vi "p2.vi"() -> ()   [LabVIEW 2023, in "d22.lvlib"]
uses:
  d22.lvlib
  AOC/AOC.lvlib
panel:
  out "size(s)":i32=375
  in  "Example":string="1,0,1~1,2,1\n0,0,2~2,0,2\n0,2,3~2,2,3\n0,0,4~0,2,4\n2,0,5~2,2,5\n0,1,6~2,1,6\n1,1,8~1,1,9"
  in  "Example":bool
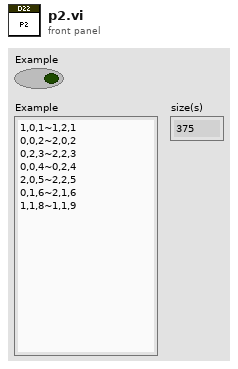
[diagram p1: front panel]
types:
  T1 = cluster{"max":cluster{"x":i32, "y":i32, "z":i32}, "min":cluster{"x":i32, "y":i32, "z":i32}, "supported by":i32[], "supporting":i32[]}
  T2 = cluster{"max":cluster{"x":i32, "y":i32, "z":i32}, "min":cluster{"x":i32, "y":i32, "z":i32}, "supported by":i32[], "supporting":i32[]}[]
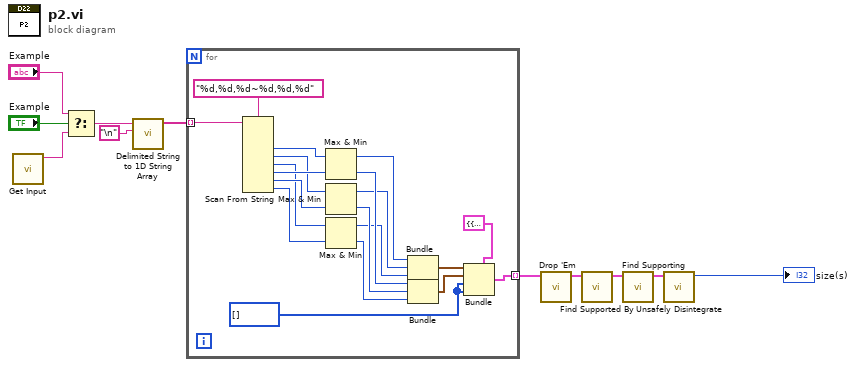
[diagram p0: block diagram]
diagram:
  n1 = call "Get Input.vi"() -> ("Input"=w11:string)  [unwired: 11 in]
  n2 = Select(t="Example", s="Example", f=w11) -> (s? t:f=w10:string)
  n3 = call <vilib>:"Delimited String to 1D String Array.vi"("delimiter"="\n", "delimited string"=w10) -> ("string array"=w7:string[])  [unwired: 9 in]
  n4 = for {
    tunnel: w7 -> [w30] mode=indexing
    tunnel: [w28] -> w6 mode=indexing
    w12 = i32[] [] ("supports")
    n5 = Scan From String(format string="%d,%d,%d~%d,%d,%d", input string=w30) -> (output 1=w26:i32, output 2=w24:i32, output 3=w22:i32, output 4=w25:i32, output 5=w23:i32, output 6=w21:i32)  [unwired: 8 in, 3 out]
    n6 = Max & Min(x=w26, y=w25) -> (max(x,y)=w16:i32, min(x,y)=w17:i32)
    n7 = Max & Min(x=w24, y=w23) -> (max(x,y)=w15:i32, min(x,y)=w18:i32)
    n8 = Max & Min(x=w22, y=w21) -> (max(x,y)=w14:i32, min(x,y)=w19:i32)
    n9 = Bundle(w16, w15, w14) -> (w29:cluster{i32, i32, i32})  [unwired: 1 in]
    n10 = Bundle(w17, w18, w19) -> (w20:cluster{i32, i32, i32})  [unwired: 1 in]
    n11 = Bundle(cluster=T1 {"max"={"x"=0, "y"=0, "z"=0}, "min"={"x"=0, "y"=0, "z"=0}, "supported by"=[], "supporting"=[]}, "max"=w29, "min"=w20, "supported by"=w12, "supporting"=w12) -> (w28:T1)
  }
  n12 = call "Drop 'Em.vi"("Bricks in"=w6) -> ("Bricks out"=w2:T2)  [unwired: 10 in]
  n13 = call "Find Supported By.vi"("Bricks in"=w2) -> ("Bricks out"=w1:T2)  [unwired: 10 in]
  n14 = call "Find Supporting.vi"("Bricks in"=w1) -> ("Bricks out"=w4:T2)  [unwired: 10 in]
  n15 = call "Unsafely Disintegrate.vi"("Bricks in"=w4) -> ("Total Disintegrated"=→"size(s)":u64)  [unwired: 10 in]
